vi "BC Async Subroutines.vi"(8 "error in (no error)":errorcluster, 11 "Bus Controller in":refnum<class "Bus Controller.lvclass">) -> (0 "error out":errorcluster, 3 "Bus Controller out":refnum<class "Bus Controller.lvclass">)   [LabVIEW 2020, in "Unit Tests.lvlib" / "Bus Controller.lvclass"]
uses:
  Bus Controller.lvclass
  <vilib>/addons/_JKI Toolkits/Caraya/classes/Test/Test.lvclass
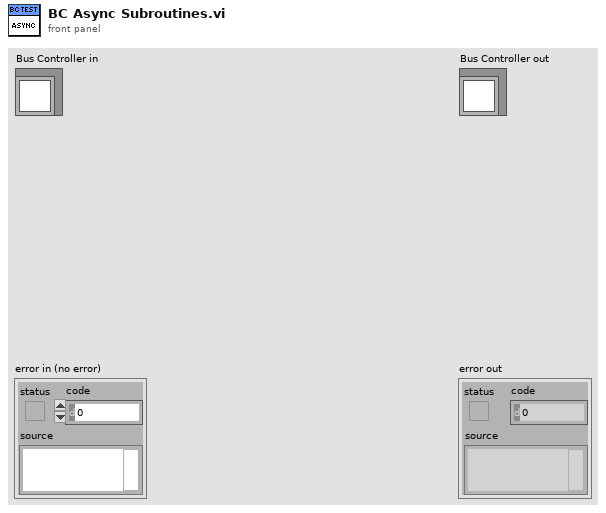
[diagram p1: front panel]
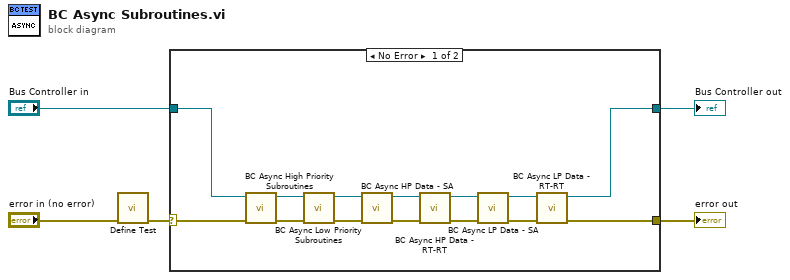
[diagram p0: block diagram]
diagram:
  n1 = call <vilib>:"Define Test.vi"("error in (no error)"="error in (no error)") -> ("error out"=w1:errorcluster)  [unwired: 9 in, 1 out]
  n2 = case shown="No Error" w1 {
    selector: w1 -> [w7 w21]
    tunnel: [w6 w21] -> w5
    tunnel: [w13 w20] -> w3
    tunnel: "Bus Controller in" -> [w19 w20]
    frame No Error {
      n3 = call "BC Async High Priority Subroutines.vi"("error in (no error)"=w7, "Bus Controller in"=w19) -> ("error out"=w12:errorcluster, "Bus Controller out"=w18:refnum<class "Bus Controller.lvclass">)  [unwired: 8 in]
      n4 = call "BC Async Low Priority Subroutines.vi"("error in (no error)"=w12, "Bus Controller in"=w18) -> ("error out"=w11:errorcluster, "Bus Controller out"=w17:refnum<class "Bus Controller.lvclass">)  [unwired: 8 in]
      n5 = call "BC Async HP Data - SA.vi"("error in (no error)"=w11, "Bus Controller in"=w17) -> ("error out"=w10:errorcluster, "Bus Controller out"=w16:refnum<class "Bus Controller.lvclass">)  [unwired: 8 in]
      n6 = call "BC Async HP Data - RT-RT.vi"("error in (no error)"=w10, "Bus Controller in"=w16) -> ("error out"=w9:errorcluster, "Bus Controller out"=w15:refnum<class "Bus Controller.lvclass">)  [unwired: 8 in]
      n7 = call "BC Async LP Data - SA.vi"("error in (no error)"=w9, "Bus Controller in"=w15) -> ("error out"=w8:errorcluster, "Bus Controller out"=w14:refnum<class "Bus Controller.lvclass">)  [unwired: 8 in]
      n8 = call "BC Async LP Data - RT-RT.vi"("error in (no error)"=w8, "Bus Controller in"=w14) -> ("error out"=w6:errorcluster, "Bus Controller out"=w13:refnum<class "Bus Controller.lvclass">)  [unwired: 8 in]
    }
    frame Error {
    }
  }
  "error out" <- w5
  "Bus Controller out" <- w3
